vi "PrintFPanel.vi"(2 "printer name (default)":string caption="Printer Name (Default)", 3 "vi name":string caption="VI Name") -> ()   [LabVIEW 2014]
uses:
  <vilib>/Utility/NIReport.llb/NI_report.lvclass
  <vilib>/Utility/NIReport.llb/NI_ReportGenerationCore.lvlib
panel:
  out "error out":errorcluster
  in  "error in (no error)":errorcluster
  # "Prints the front panel of a VI"
  # "The named VI must already be in memory !!"
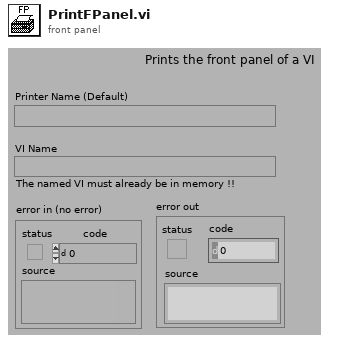
[diagram p1: front panel]
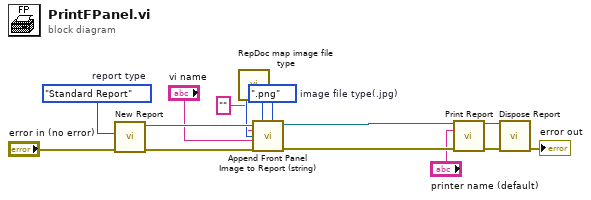
[diagram p0: block diagram]
diagram:
  w7 = enum16{"Standard Report", "HTML"}."Standard Report"  # report type
  w8 = enum16{".jpg", ".png"}.".png"  # image file type(.jpg)
  n1 = call <vilib>:"New Report.vi"("report type"=w7, "error in (no error)"="error in (no error)") -> ("report out"=w13:refnum<class "NI_report.lvclass">, "error out"=w14:errorcluster)  [unwired: 12 in]
  n2 = call <vilib>:"RepDoc map image file type.vi"("image file type (.jpg)"=w8) -> ("image format (jpeg)"=w2:enum32{"PNG", "JPEG", "GIF"})
  n3 = call <vilib>:"Append Front Panel Image to Report (string).vi"("report in"=w13, "image format (jpeg)"=w2, "VI"="", "description"="vi name", "error in (no error)"=w14) -> ("report out"=w11:refnum<class "NI_report.lvclass">, "error out"=w12:errorcluster)  [unwired: 6 in, 3 out]
  n4 = call-dynamic "Print Report.vi"("report in"=w11, "printer name (default)"="printer name (default)", "error in (no error)"=w12) -> ("report out"=w10:refnum<class "NI_report.lvclass">, "error out"=w9:errorcluster)  [unwired: 11 in]
  n5 = call-dynamic "Dispose Report.vi"("report in"=w10, "error in (no error)"=w9) -> ("error out"=→"error out":errorcluster)  [unwired: 13 in]
